vi "Get Voltage.vi"(0 "reference in":refnum<class "Power Supply.lvclass">, 5 "error in (no error)":errorcluster) -> (14 "reference out":refnum<class "Power Supply.lvclass">, 17 "Power Supply Voltage Setting":dbl, 18 "Power Supply Voltage Reading":dbl, 19 "error out":errorcluster)   [LabVIEW 2017, in "Power Supply.lvclass"]
uses:
  Power Supply.lvclass
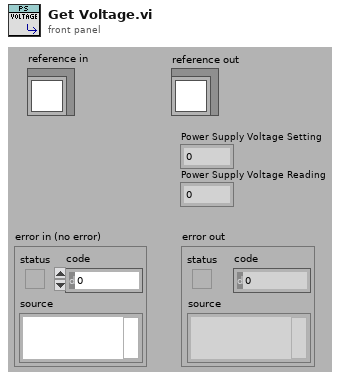
[diagram p1: front panel]
types:
  T1 = typedef "Power Supply.lvclass/ObjectAttributes.ctl" = cluster{"Power Supply Chain VISA Session":refnum<visa-resource-name>, "Power Supply Chain Address":i16, "Power Supply Open/Close Status":bool, "Power Supply Voltage Setting":dbl, "Power Supply Current Setting":dbl, "Power Supply Voltage Reading":dbl, "Power Supply Current Reading":dbl, "Power Supply Status":T2, "Power Supply Error":T3, "Fault Register":u8, "Power Supply Error":bool}
  T2 = typedef "Power Supply.lvclass/Power Supply Status.ctl" = enum16{"Closed", "Open"}
  T3 = typedef "Power Supply.lvclass/Power Supply Error.ctl" = enum16{"None", "Read Error"}
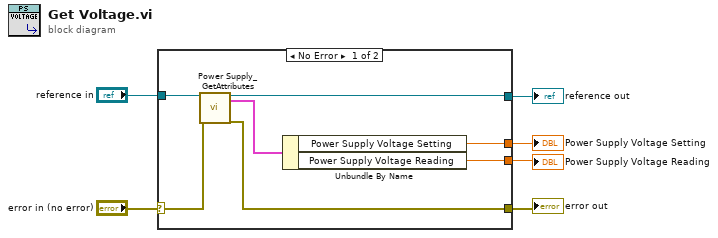
[diagram p0: block diagram]
diagram:
  n1 = case shown="No Error" "error in (no error)" {
    selector: "error in (no error)" -> [w12 w15]
    tunnel: [w9 w15] -> w5
    tunnel: [w10 w14] -> w3
    tunnel: "reference in" -> [w13 w14]
    tunnel: [w8 _] -> w2
    tunnel: [w7 _] -> w1
    frame No Error {
      n2 = call "Power Supply_GetAttributes.vi"("reference in"=w13, "error in (no error)"=w12) -> ("reference out"=w10:refnum<class "Power Supply.lvclass">, "Data"=w11:T1, "error out"=w9:errorcluster)  [unwired: 14 in, 1 out]
      n3 = Unbundle By Name(w11) -> ("Power Supply Voltage Setting"=w7:dbl, "Power Supply Voltage Reading"=w8:dbl)
    }
    frame Error {
    }
  }
  "error out" <- w5
  "reference out" <- w3
  "Power Supply Voltage Setting" <- w1
  "Power Supply Voltage Reading" <- w2
